vi "Distance Logger.vi"() -> ()   [LabVIEW 2011]
uses:
  Robot Global Data.vi
panel:
  out "Distance to Target":dbl[](graph)
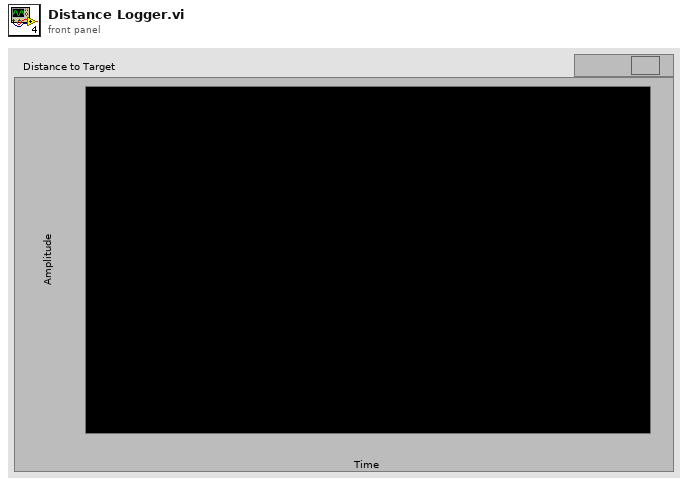
[diagram p1: front panel]
types:
  T1 = enum16{"open", "replace", "create", "open or create", "replace or create", "replace or create with confirmation"}
  T2 = cluster{"Position":cluster{"X":dbl, "Y":dbl}, "Distance (ft)":dbl}[]
  T3 = cluster{"Position":cluster{"X":dbl, "Y":dbl}, "Distance (ft)":dbl}
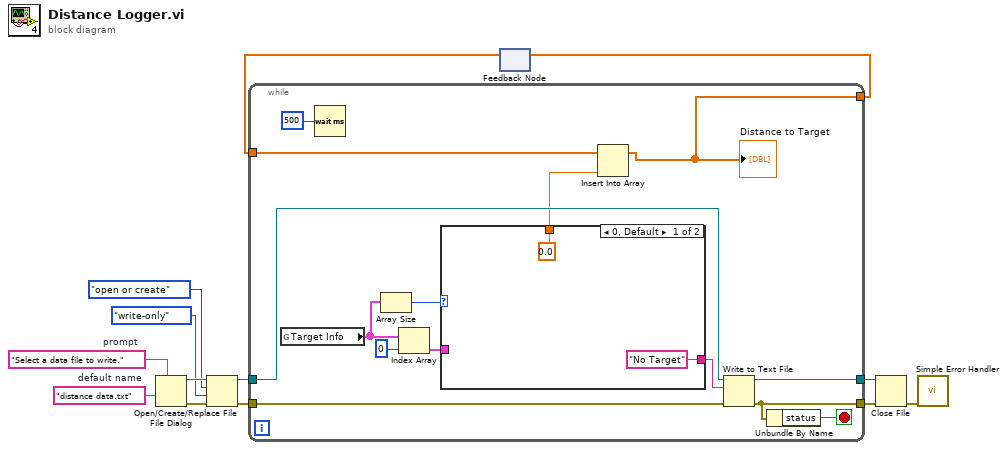
[diagram p0: block diagram]
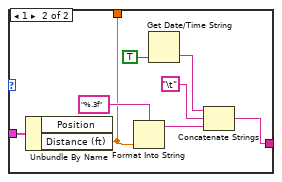
[diagram p2: hidden frame]
diagram:
  w12 = "distance data.txt"  # default name
  w11 = "Select a data file to write."  # prompt
  n1 = File Dialog(7:w11, 9:w12) -> (0:w10:errorcluster, 3:w13:path)  [unwired: 1 in, 6 out]
  n2 = Open/Create/Replace File(file path (use dialog)=w13, error in=w10, operation (0:open)=T1."open or create", access (0:read/write)=enum16{"read/write", "read-only", "write-only"}."write-only") -> (refnum out=w7:refnum<file>, error out=w6:errorcluster)  [unwired: 3 out]
  n3 = feedback #1() -> (w1:dbl[])  [unwired: 1 in]
  n4 = while {
    tunnel: w7 -> [w27]
    tunnel: w6 -> [w26]
    tunnel: [w25] -> w4
    tunnel: [w21] -> w3
    tunnel: [w15] -> w2
    tunnel: w1 -> [w14]
    stop <- w20 stop-if-true
    n5 = global read "Robot Global Data.vi" "Target Info"() -> (w19:T2)
    n6 = Wait (ms)(milliseconds to wait=u32 500 ("millisecond multiple")) -> ()  [unwired: 1 out]
    n7 = Array Size(array=w19) -> (size(s)=w23:i32)
    n8 = Index Array(array=w19, index=0) -> (element=w17:T3)
    n9 = case shown="0, Default" w23 {
      tunnel: ["No Target" w31] -> w22
      tunnel: w17 -> [_ w37]
      tunnel: [0.0 ("Distance (ft)") w30] -> w16
      frame 0, Default {
      }
      frame 1 {
        n10 = Unbundle By Name(w37) -> ("Distance (ft)"=w30:dbl)  [unwired: 1 out]
        n11 = Format Into String(format string="%.3f", w30) -> (resulting string=w32:string)  [unwired: 2 in, 1 out]
        n12 = Get Date/Time String(want seconds? (F)=TRUE) -> (time string=w34:string)  [unwired: 2 in, 1 out]
        n13 = Concatenate Strings(w34, "\t", w32) -> (w31:string)
      }
    }
    n14 = Insert Into Array(array=w14, new element=w16) -> (w15:dbl[])  [unwired: 1 in]
    "Distance to Target" <- w15
    n15 = Write to Text File(file (use dialog)=w27, text=w22, error in=w26) -> (refnum out=w25:refnum<file>, error out=w21:errorcluster)  [unwired: 1 in, 1 out]
    n16 = Unbundle By Name(w21) -> ("status"=w20:bool)
  }
  n17 = feedback-in #1(w2) -> ()
  n18 = Close File(refnum=w4, error in=w3) -> (error out=w5:errorcluster)  [unwired: 1 out]
  n19 = call <vilib>:"Simple Error Handler.vi"("error in (no error)"=w5) -> ()  [unwired: 1 in, 8 out]
